vi "Generate Address Frame Vectors.vi"(0 "RFFE Extended Command in":refnum<class "RFFE Extended Command.lvclass">, 11 "error in (no error)":errorcluster) -> (4 "RFFE Extended Command out":refnum<class "RFFE Extended Command.lvclass">, 6 "Address Frame Vectors":string[](array[string]), 15 "error out":errorcluster)   [LabVIEW 2018, in "MIPI RFFE API.lvlib" / "RFFE Extended Command.lvclass"]
uses:
  RFFE Extended Command.lvclass
  MIPI RFFE API.lvlib
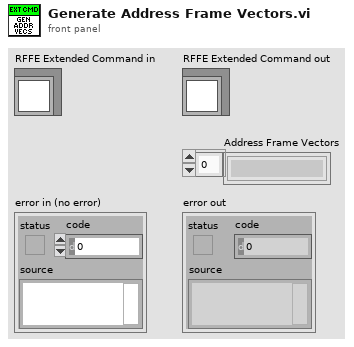
[diagram p1: front panel]
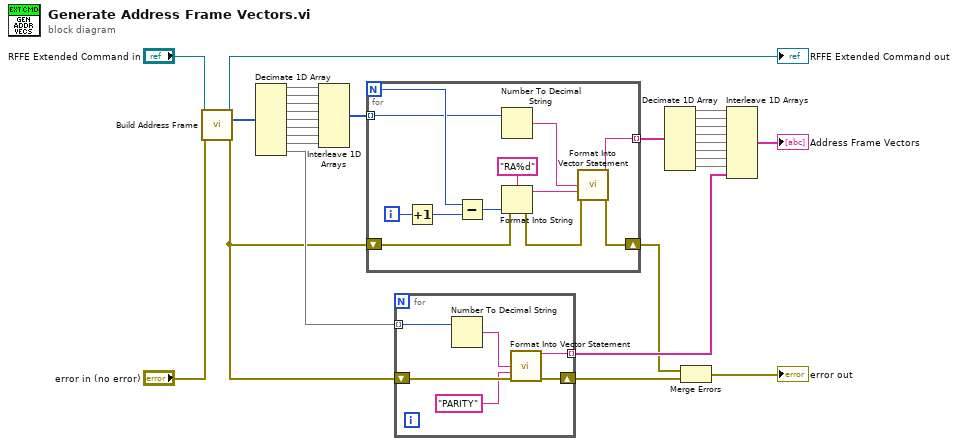
[diagram p0: block diagram]
diagram:
  n1 = call-dynamic "Build Address Frame.vi"("RFFE Extended Command in"="RFFE Extended Command in", "error in (no error)"="error in (no error)") -> ("RFFE Extended Command out"=→"RFFE Extended Command out":refnum<class "RFFE Extended Command.lvclass">, "Address Frame"=w1:u8[], "error out"=w5:errorcluster)  [unwired: 11 in]
  n2 = Decimate 1D Array(w1) -> (w19:u8[], w20:u8[], w21:u8[], w22:u8[], w23:u8[], w24:u8[], w25:u8[], w26:u8[], w17:u8[])
  n3 = Interleave 1D Arrays(w19, w20, w21, w22, w23, w24, w25, w26) -> (w18:u8[])
  n4 = for {
    N -> [w41]
    tunnel: w18 -> [w35] mode=indexing
    shift-right: [w36] -> w3
    shift-left: w5 -> [w31]
    tunnel: [w33] -> w16 mode=indexing
    i -> [w39]
    n5 = Increment(x=w39) -> (x+1=w40:i32)
    n6 = Subtract(x=w41, y=w40) -> (x-y=w38:i32)
    n7 = Number To Decimal String(number=w35) -> (decimal integer string=w34:string)  [unwired: 1 in]
    n8 = Format Into String(format string="RA%d", error in=w31, w38) -> (resulting string=w37:string, error out=w30:errorcluster)  [unwired: 1 in]
    n9 = call "Format Into Vector Statement.vi"("DATA (0)"=w34, "Comment"=w37, "error in (no error)"=w30) -> ("Vector Statement"=w33:string, "error out"=w36:errorcluster)  [unwired: 11 in]
  }
  n10 = for {
    shift-right: [w45] -> w4
    shift-left: w5 -> [w46]
    tunnel: w17 -> [w43] mode=indexing
    tunnel: [w42] -> w6 mode=indexing
    n11 = Number To Decimal String(number=w43) -> (decimal integer string=w47:string)  [unwired: 1 in]
    n12 = call "Format Into Vector Statement.vi"("DATA (0)"=w47, "Comment"="PARITY", "error in (no error)"=w46) -> ("Vector Statement"=w42:string, "error out"=w45:errorcluster)  [unwired: 11 in]
  }
  n13 = Decimate 1D Array(w16) -> (w15:string[], w14:string[], w13:string[], w12:string[], w11:string[], w10:string[], w9:string[], w8:string[])
  n14 = Merge Errors(w3, w4) -> (→"error out":errorcluster)
  n15 = Interleave 1D Arrays(w15, w14, w13, w12, w11, w10, w9, w8, w6) -> (→"Address Frame Vectors":string[])
